vi "ni579x Erase EEPROM Sector.vi"(0 "Register Bus":refnum<class "ni579x Register Bus v1 Host.lvclass">=refnum, 1 "scope":string(combo)="characterization data eeprom", 11 "Error In":errorcluster) -> (4 "Register Bus (out)":refnum<class "ni579x Register Bus v1 Host.lvclass">, 15 "Error Out":errorcluster)   [LabVIEW 2015]
uses:
  <instrlib>/ni579x/Register Bus/v1/Host/ni579x Register Bus v1 Host.lvclass
  <instrlib>/ni579x/Config/v1/Shared/Types/ni579x FAM Register Offset.ctl
  <instrlib>/ni579x/Config/v1/Shared/Types/ni579x FAM Register Operation.ctl
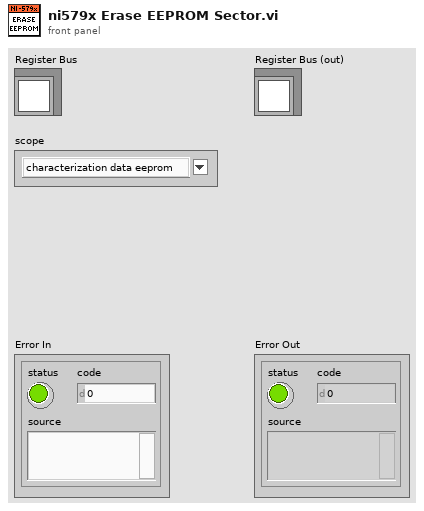
[diagram p1: front panel]
types:
  T1 = typedef "ni579x FAM Register Operation.ctl" = cluster{"FAM Register Offset":T2, "Address":u32, "Write (T)/Read (F)":bool, "Write Data":u32}
  T2 = typedef "ni579x FAM Register Offset.ctl" = u8
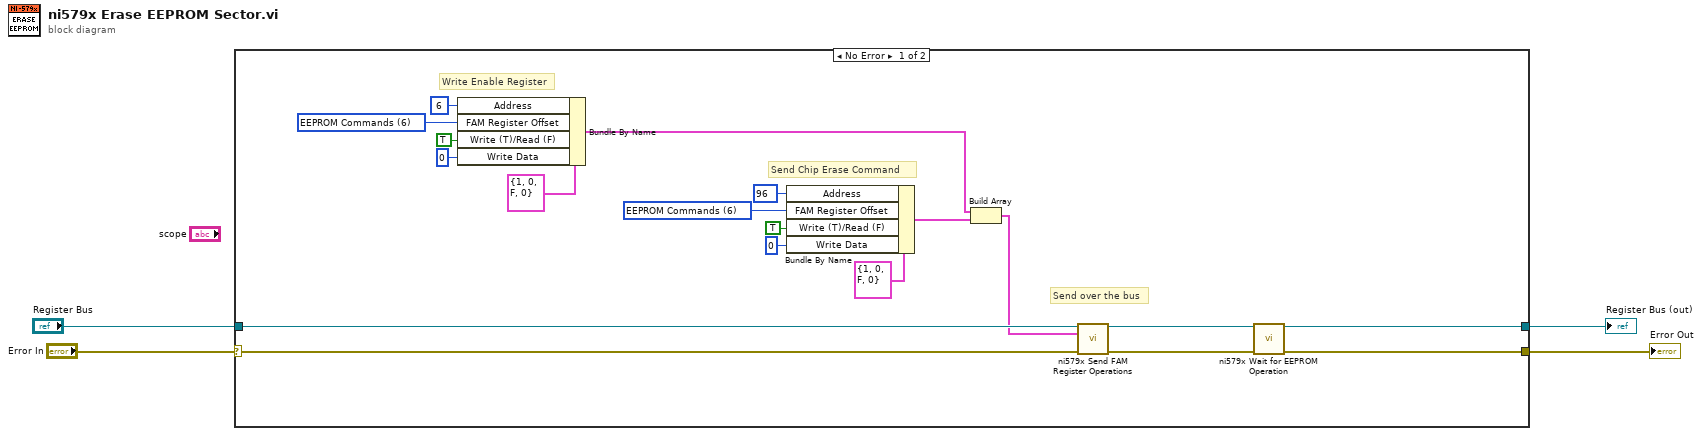
[diagram p0: block diagram]
diagram:
  n1 = case shown="No Error" "Error In" {
    selector: "Error In" -> [w22 w25]
    tunnel: [w9 w25] -> w3
    tunnel: "Register Bus" -> [w23 w24]
    tunnel: [w10 w24] -> w1
    frame No Error {
      w6 = T2 6 items=["ADC"=1, "DAC"=2, "Clock Distribution Chip"=3, "Frequency/Phase Adjust DAC"=4, "EEPROM"=5, "EEPROM Commands"=6, "LO1"=7, "Rx Atten Pre-LNA"=9, "Rx Atten Post-LNA"=10, "Tx Atten"=11] ("FAM Register Offset")
      w8 = T2 6 items=["ADC"=1, "DAC"=2, "Clock Distribution Chip"=3, "Frequency/Phase Adjust DAC"=4, "EEPROM"=5, "EEPROM Commands"=6, "LO1"=7, "Rx Atten Pre-LNA"=9, "Rx Atten Post-LNA"=10, "Tx Atten"=11] ("FAM Register Offset")
      # "Write Enable Register"
      # "Send Chip Erase Command"
      # "Send over the bus"
      n2 = Bundle By Name(cluster=T1 {"FAM Register Offset"=1, "Address"=0, "Write (T)/Read (F)"=FALSE, "Write Data"=0} ("FAM Register Operation"), "Address"=u32 6, "FAM Register Offset"=w8, "Write (T)/Read (F)"=TRUE, "Write Data"=u32 0) -> (w13:T1)
      n3 = Bundle By Name(cluster=T1 {"FAM Register Offset"=1, "Address"=0, "Write (T)/Read (F)"=FALSE, "Write Data"=0} ("FAM Register Operation"), "Address"=u32 96, "FAM Register Offset"=w6, "Write (T)/Read (F)"=TRUE, "Write Data"=u32 0) -> (w18:T1)
      n4 = Build Array(w13, w18) -> (w17:T1[])
      n5 = call <instrlib>:"ni579x Send FAM Register Operations.vi"("Register Bus"=w23, "FAM Register Operations"=w17, "Error In"=w22) -> ("Register Bus (out)"=w11:refnum<class "ni579x Register Bus v1 Host.lvclass">, "Error Out"=w12:errorcluster)  [unwired: 10 in, 1 out]
      n6 = call <instrlib>:"ni579x Wait for EEPROM Operation.vi"("Register Bus"=w11, "Error In"=w12) -> ("Register Bus (out)"=w10:refnum<class "ni579x Register Bus v1 Host.lvclass">, "Error Out"=w9:errorcluster)  [unwired: 12 in]
    }
    frame Error {
    }
  }
  "Register Bus (out)" <- w1
  "Error Out" <- w3
